vi "EL6995.vi"(8 "error in (no error)":errorcluster, 11 "EL6695UserOutputs":T3) -> (0 "error out":errorcluster, 1 "Read Status":bool[](array[boolean]), 2 "EL6695UserInputs":T1, 3 "EL6695DefaultInputs":T2, 10 "Write Status":bool[](array[boolean]))   [LabVIEW 2022 SP3, in "IO_Library.lvlib"]
doc: "VI implementing the EL6695.\n\nBlock reads and writes to a terminal.\n\nTo use, modify the constant string entering the ADS Init block with your string (created with the ADS Path Helper). \n\nThe EL6695 requires additional configuration based on the configured inputs/outputs in the linked TwinCAT project. These can be modified firstly in the type definitions for user inputs and outputs, then inside this vi, modify the variant to cluster converters (only the User ones)."
uses:
  IO_Library.lvlib
  TypeDefs/EL6695UserOutputs.ctl
  TypeDefs/EL6695DefaultInputs.ctl
  TypeDefs/EL6695UserInputs.ctl
  ADS/ADS_Library.lvlib
panel:
  out "bHasMatched":bool[](array[boolean])
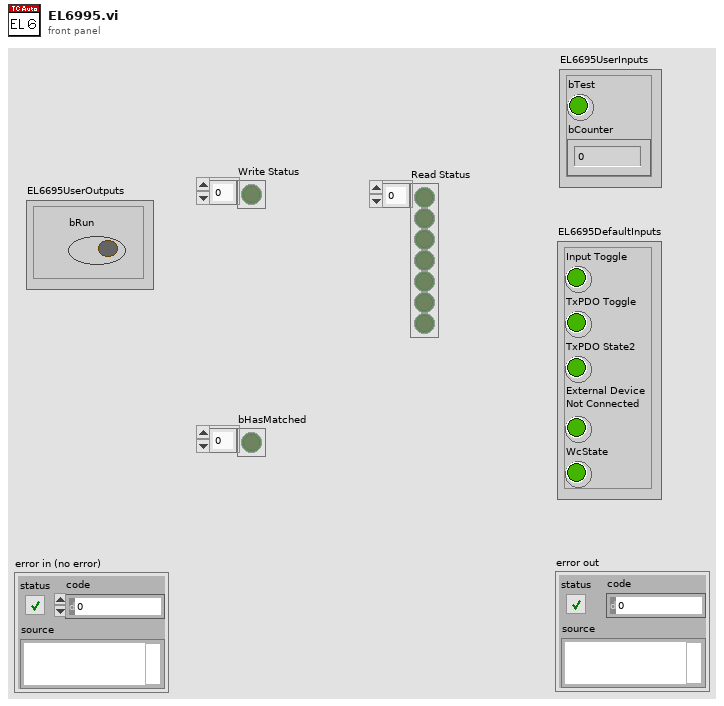
[diagram p1: front panel]
types:
  T1 = typedef "IO_Library.lvlib/EL6695UserInputs.ctl" = cluster{"bTest":bool, "bCounter":dbl}
  T2 = typedef "IO_Library.lvlib/EL6695DefaultInputs.ctl" = cluster{"Input Toggle":bool, "TxPDO Toggle":bool, "TxPDO State2":bool, "External Device \nNot Connected":bool, "WcState":bool}
  T3 = typedef "IO_Library.lvlib/EL6695UserOutputs.ctl" = cluster{"bRun":bool}
  T4 = cluster{"[0]":variant, "[1]":variant, "[2]":variant, "[3]":variant, "[4]":variant, "[5]":variant, "[6]":variant}
  T5 = cluster{"[0]":variant, "[1]":variant, "[2]":variant, "[3]":variant, "[4]":variant}
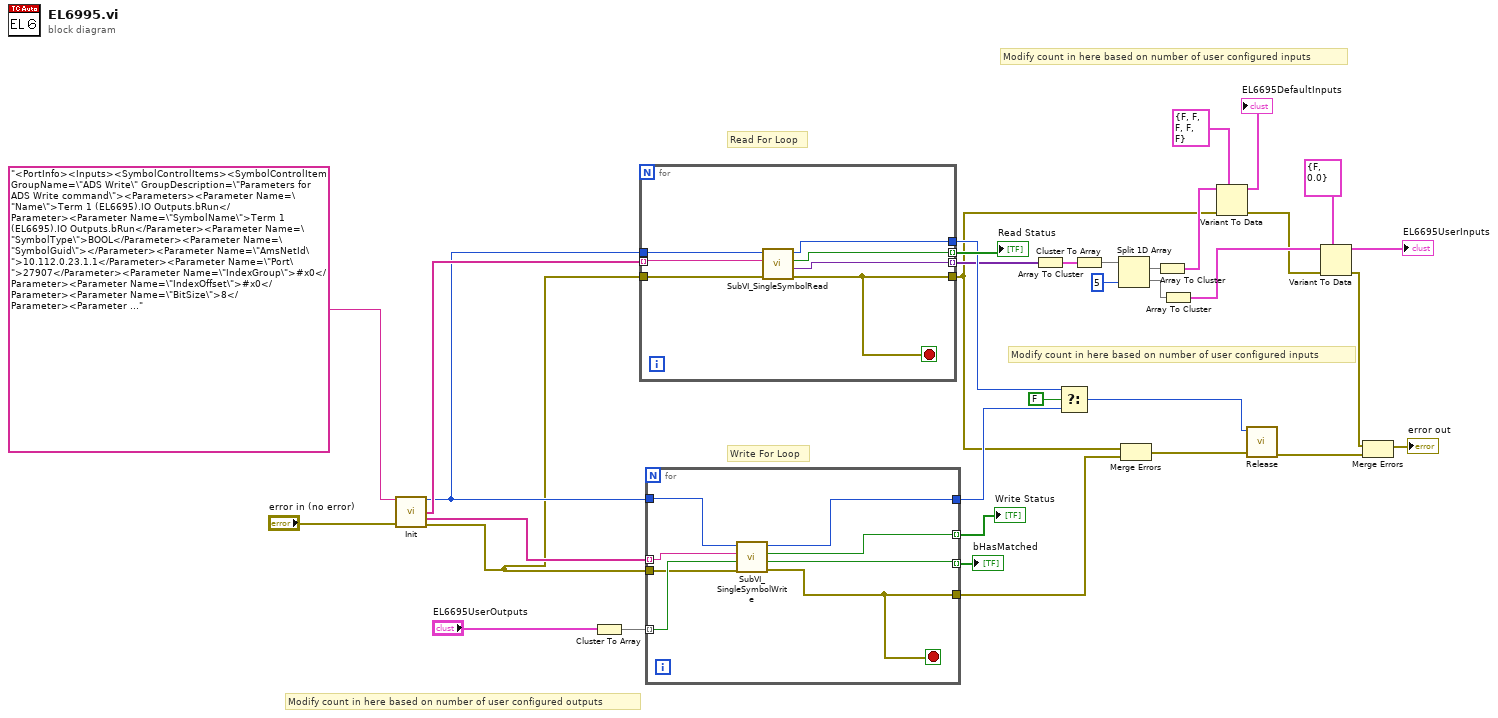
[diagram p0: block diagram]
diagram:
  # "Modify count in here based on number of user configured outputs"
  # "Modify count in here based on number of user configured inputs"
  # "Modify count in here based on number of user configured inputs"
  # "Read For Loop"
  # "Write For Loop"
  n1 = call <userlib>:"Init.vi"("XMLDescription"="<PortInfo><Inputs><SymbolControlItems><SymbolControlItem GroupName=\"ADS Write\" GroupDescription=\"Parameters for ADS Write command\"><Parameters><Parameter Name=\"Name\">Term 1 (EL6695).IO Outputs.bRun</Parameter><Parameter Name=\"SymbolName\">Term 1 (EL6695).IO Outputs.bRun</Parameter><Parameter Name=\"SymbolType\">BOOL</Parameter><Parameter Name=\"SymbolGuid\"></Parameter><Parameter Name=\"AmsNetId\">10.112.0.23.1.1</Parameter><Parameter Name=\"Port\">27907</Parameter><Parameter Name=\"IndexGroup\">#x0</Parameter><Parameter Name=\"IndexOffset\">#x0</Parameter><Parameter Name=\"BitSize\">8</Parameter><Parameter Name=\"CycleTime [ms]\">10</Parameter><Parameter Name=\"Timeout [ms]\">1000</Parameter></Parameters></SymbolControlItem></SymbolControlItems></Inputs><Outputs><SymbolControlItems><SymbolControlItem GroupName=\"ADS Read\" GroupDescription=\"Parameters for ADS Read command\"><Parameters><Parameter Name=\"Name\">Term 1 (EL6695).InputToggle</Parameter><Parameter Name=\"SymbolName\">Term 1 (EL6695).InputToggle</Parameter><Parameter Name=\"SymbolType\">BIT</Parameter><Parameter Name=\"SymbolGuid\"></Parameter><Parameter Name=\"AmsNetId\">10.112.0.23.1.1</Parameter><Parameter Name=\"Port\">27907</Parameter><Parameter Name=\"IndexGroup\">#x0</Parameter><Parameter Name=\"IndexOffset\">#x0</Parameter><Parameter Name=\"BitSize\">1</Parameter><Parameter Name=\"CycleTime [ms]\">10</Parameter><Parameter Name=\"Transmode\">3</Parameter><Parameter Name=\"Timeout [ms]\">1000</Parameter><Parameter Name=\"TCBufferSize [Samples]\">10</Parameter><Parameter Name=\"LVBufferSize [Samples]\">50</Parameter><Parameter Name=\"Expected min delay [ms]\">500</Parameter></Parameters></SymbolControlItem><SymbolControlItem GroupName=\"ADS Read\" GroupDescription=\"Parameters for ADS Read command\"><Parameters><Parameter Name=\"Name\">Term 1 (EL6695).SYNC Inputs.TxPDO toggle</Parameter><Parameter Name=\"SymbolName\">Term 1 (EL6695).SYNC Inputs.TxPDO toggle</Parameter><Parameter Name=\"SymbolType\">BIT</Parameter><Parameter Name=\"SymbolGuid\"></Parameter><Parameter Name=\"AmsNetId\">10.112.0.23.1.1</Parameter><Parameter Name=\"Port\">27907</Parameter><Parameter Name=\"IndexGroup\">#x0</Parameter><Parameter Name=\"IndexOffset\">#x0</Parameter><Parameter Name=\"BitSize\">1</Parameter><Parameter Name=\"CycleTime [ms]\">10</Parameter><Parameter Name=\"Transmode\">3</Parameter><Parameter Name=\"Timeout [ms]\">1000</Parameter><Parameter Name=\"TCBufferSize [Samples]\">10</Parameter><Parameter Name=\"LVBufferSize [Samples]\">50</Parameter><Parameter Name=\"Expected min delay [ms]\">500</Parameter></Parameters></SymbolControlItem><SymbolControlItem GroupName=\"ADS Read\" GroupDescription=\"Parameters for ADS Read command\"><Parameters><Parameter Name=\"Name\">Term 1 (EL6695).SYNC Inputs.TxPDO state</Parameter><Parameter Name=\"SymbolName\">Term 1 (EL6695).SYNC Inputs.TxPDO state</Parameter><Parameter Name=\"SymbolType\">BIT</Parameter><Parameter Name=\"SymbolGuid\"></Parameter><Parameter Name=\"AmsNetId\">10.112.0.23.1.1</Parameter><Parameter Name=\"Port\">27907</Parameter><Parameter Name=\"IndexGroup\">#x0</Parameter><Parameter Name=\"IndexOffset\">#x0</Parameter><Parameter Name=\"BitSize\">1</Parameter><Parameter Name=\"CycleTime [ms]\">10</Parameter><Parameter Name=\"Transmode\">3</Parameter><Parameter Name=\"Timeout [ms]\">1000</Parameter><Parameter Name=\"TCBufferSize [Samples]\">10</Parameter><Parameter Name=\"LVBufferSize [Samples]\">50</Parameter><Parameter Name=\"Expected min delay [ms]\">500</Parameter></Parameters></SymbolControlItem><SymbolControlItem GroupName=\"ADS Read\" GroupDescription=\"Parameters for ADS Read command\"><Parameters><Parameter Name=\"Name\">Term 1 (EL6695).SYNC Inputs.External device not connected</Parameter><Parameter Name=\"SymbolName\">Term 1 (EL6695).SYNC Inputs.External device not connected</Parameter><Parameter Name=\"SymbolType\">BIT</Parameter><Parameter Name=\"SymbolGuid\"></Parameter><Parameter Name=\"AmsNetId\">10.112.0.23.1.1</Parameter><Parameter Name=\"Port\">27907</Parameter><Parameter Name=\"IndexGroup\">#x0</Parameter><Parameter Name=\"IndexOffset\">#x0</Parameter><Parameter Name=\"BitSize\">1</Parameter><Parameter Name=\"CycleTime [ms]\">10</Parameter><Parameter Name=\"Transmode\">3</Parameter><Parameter Name=\"Timeout [ms]\">1000</Parameter><Parameter Name=\"TCBufferSize [Samples]\">10</Parameter><Parameter Name=\"LVBufferSize [Samples]\">50</Parameter><Parameter Name=\"Expected min delay [ms]\">500</Parameter></Parameters></SymbolControlItem><SymbolControlItem GroupName=\"ADS Read\" GroupDescription=\"Parameters for ADS Read command\"><Parameters><Parameter Name=\"Name\">Term 1 (EL6695).WcState</Parameter><Parameter Name=\"SymbolName\">Term 1 (EL6695).WcState</Parameter><Parameter Name=\"SymbolType\">BIT</Parameter><Parameter Name=\"SymbolGuid\"></Parameter><Parameter Name=\"AmsNetId\">10.112.0.23.1.1</Parameter><Parameter Name=\"Port\">27907</Parameter><Parameter Name=\"IndexGroup\">#x0</Parameter><Parameter Name=\"IndexOffset\">#x0</Parameter><Parameter Name=\"BitSize\">1</Parameter><Parameter Name=\"CycleTime [ms]\">10</Parameter><Parameter Name=\"Transmode\">3</Parameter><Parameter Name=\"Timeout [ms]\">1000</Parameter><Parameter Name=\"TCBufferSize [Samples]\">10</Parameter><Parameter Name=\"LVBufferSize [Samples]\">50</Parameter><Parameter Name=\"Expected min delay [ms]\">500</Parameter></Parameters></SymbolControlItem><SymbolControlItem GroupName=\"ADS Read\" GroupDescription=\"Parameters for ADS Read command\"><Parameters><Parameter Name=\"Name\">Term 1 (EL6695).IO Inputs.bTest</Parameter><Parameter Name=\"SymbolName\">Term 1 (EL6695).IO Inputs.bTest</Parameter><Parameter Name=\"SymbolType\">BOOL</Parameter><Parameter Name=\"SymbolGuid\"></Parameter><Parameter Name=\"AmsNetId\">10.112.0.23.1.1</Parameter><Parameter Name=\"Port\">27907</Parameter><Parameter Name=\"IndexGroup\">#x0</Parameter><Parameter Name=\"IndexOffset\">#x0</Parameter><Parameter Name=\"BitSize\">8</Parameter><Parameter Name=\"CycleTime [ms]\">10</Parameter><Parameter Name=\"Transmode\">3</Parameter><Parameter Name=\"Timeout [ms]\">1000</Parameter><Parameter Name=\"TCBufferSize [Samples]\">10</Parameter><Parameter Name=\"LVBufferSize [Samples]\">50</Parameter><Parameter Name=\"Expected min delay [ms]\">500</Parameter></Parameters></SymbolControlItem><SymbolControlItem GroupName=\"ADS Read\" GroupDescription=\"Parameters for ADS Read command\"><Parameters><Parameter Name=\"Name\">Term 1 (EL6695).IO Inputs.bCounter</Parameter><Parameter Name=\"SymbolName\">Term 1 (EL6695).IO Inputs.bCounter</Parameter><Parameter Name=\"SymbolType\">INT</Parameter><Parameter Name=\"SymbolGuid\"></Parameter><Parameter Name=\"AmsNetId\">10.112.0.23.1.1</Parameter><Parameter Name=\"Port\">27907</Parameter><Parameter Name=\"IndexGroup\">#x0</Parameter><Parameter Name=\"IndexOffset\">#x0</Parameter><Parameter Name=\"BitSize\">16</Parameter><Parameter Name=\"CycleTime [ms]\">10</Parameter><Parameter Name=\"Transmode\">3</Parameter><Parameter Name=\"Timeout [ms]\">1000</Parameter><Parameter Name=\"TCBufferSize [Samples]\">10</Parameter><Parameter Name=\"LVBufferSize [Samples]\">50</Parameter><Parameter Name=\"Expected min delay [ms]\">500</Parameter></Parameters></SymbolControlItem></SymbolControlItems></Outputs></PortInfo>", "error in (no error)"="error in (no error)") -> ("Handle"=w27:u32, "ReadGrpSymbols"=w28:string[], "WriteGrpSymbols"=w31:string[], "error out"=w26:errorcluster)  [unwired: 9 in, 1 out]
  n2 = Cluster To Array(cluster="EL6695UserOutputs") -> (array=w32:bool[])
  n3 = for {
    tunnel: w28 -> [w41] mode=indexing
    tunnel: w27 -> [w40]
    tunnel: w26 -> [w39]
    tunnel: [w38] -> w6
    tunnel: [w36] -> w23 mode=indexing
    tunnel: [w37] -> w16 mode=indexing
    tunnel: [w35] -> w21
    stop <- w38 stop-if-true
    n4 = call "SubVI_SingleSymbolRead.vi"("error in (no error)"=w39, "SymbolName"=w41, "Handle In"=w40) -> ("error out"=w38:errorcluster, "RData"=w37:variant, "Read status?"=w36:bool, "Handle Out"=w35:u32)  [unwired: 5 in]
  }
  "Read Status" <- w23
  n5 = for {
    tunnel: w32 -> [w47] mode=indexing
    tunnel: w31 -> [w48] mode=indexing
    tunnel: w26 -> [w46]
    tunnel: w27 -> [w49]
    tunnel: [w42] -> w25
    tunnel: [w44] -> w29 mode=indexing
    tunnel: [w45] -> w30 mode=indexing
    tunnel: [w43] -> w22
    stop <- w42 stop-if-true
    n6 = call "SubVI_SingleSymbolWrite.vi"("error in"=w46, "WData"=w47, "SymbolName"=w48, "Handle In"=w49) -> ("error out"=w42:errorcluster, "bHasMatched"=w44:bool, "Write Status"=w45:bool, "Handle Out"=w43:u32)  [unwired: 4 in]
  }
  "bHasMatched" <- w29
  "Write Status" <- w30
  n7 = Array To Cluster(array=w16) -> (cluster=w13:T4)
  n8 = Select(t=w21, s=FALSE, f=w22) -> (s? t:f=w19:u32)
  n9 = Cluster To Array(cluster=w13) -> (array=w12:variant[])
  n10 = Split 1D Array(array=w12, index=5) -> (first subarray=w10:variant[], second subarray=w5:variant[])
  n11 = Merge Errors(w6, w25) -> (w24:errorcluster)
  n12 = Array To Cluster(array=w10) -> (cluster=w9:T5)
  n13 = Array To Cluster(array=w5) -> (cluster=w7:cluster{"[0]":variant, "[1]":variant})
  n14 = Variant To Data(error in=w6, type=T2 {"Input Toggle"=FALSE, "TxPDO Toggle"=FALSE, "TxPDO State2"=FALSE, "External Device \nNot Connected"=FALSE, "WcState"=FALSE} ("EL6695DefaultInputs"), Variant=w9) -> (data=→"EL6695DefaultInputs":T2, error out=w4:errorcluster)
  n15 = call <userlib>:"Release.vi"("Handle"=w19, "error in (no error)"=w24) -> ("error out"=w17:errorcluster)  [unwired: 13 in]
  n16 = Variant To Data(error in=w4, type=T1 {"bTest"=FALSE, "bCounter"=0.0} ("EL6695UserInputs"), Variant=w7) -> (data=→"EL6695UserInputs":T1, error out=w1:errorcluster)
  n17 = Merge Errors(w1, w17) -> (→"error out":errorcluster)
